vi "Get Package Installed Version.vi"(8 "error in":errorcluster, 11 "package name":string) -> (0 "error out":errorcluster, 1 "installed?":bool, 2 "installed version":string, 3 "package name out":string)   [LabVIEW 2014, in "NIPM_API.lvlib"]
doc: "Returns the version of the package that is currently installed.\n\nINPUT(s)\n<B>Package name</B>: Specifies the package\n\nOUTPUT(s)\n<B>Package name out</B>: Outputs the package name\n\n<B>Installed version</B>: Outputs the currently installed version of the package\n\n<B>Installed?</B>: Outputs whether or not the package is currently installed"
uses:
  NIPM_API.lvlib
panel:
  out "cmd standard output":string
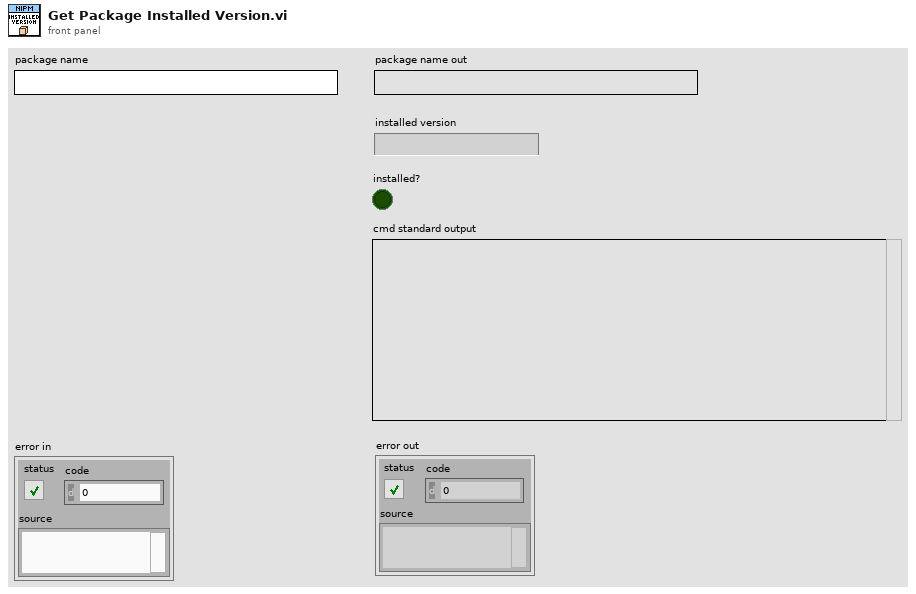
[diagram p1: front panel]
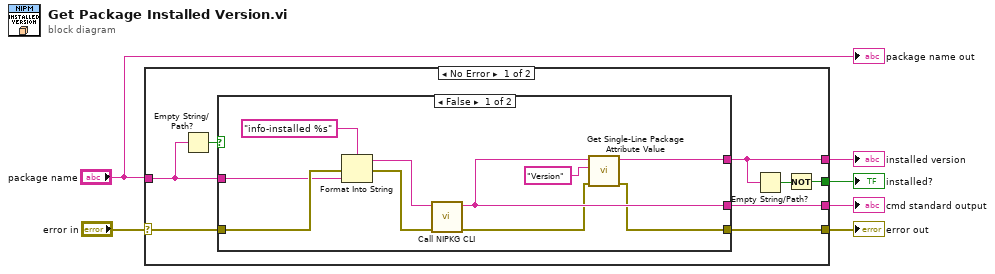
[diagram p0: block diagram]
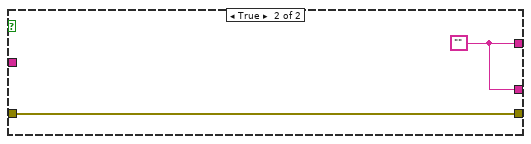
[diagram p2: hidden frame]
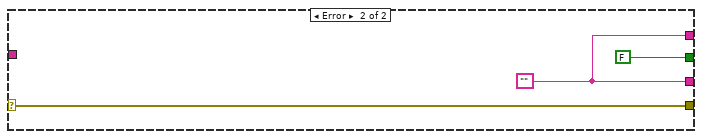
[diagram p3: hidden frame]
diagram:
  n1 = case shown="No Error" "error in" {
    selector: "error in" -> [w14 w29]
    tunnel: [w13 w28] -> w5
    tunnel: [w12 w29] -> w4
    tunnel: "package name" -> [w11 _]
    tunnel: [w9 w28] -> w2
    tunnel: [w7 FALSE] -> w1
    frame No Error {
      n2 = Empty String/Path?(string/path=w11) -> (empty?=w10:bool)
      n3 = case shown="False" w10 {
        tunnel: w14 -> [w23 w26]
        tunnel: [w20 w25] -> w13
        tunnel: [w18 w25] -> w9
        tunnel: [w16 w26] -> w12
        tunnel: w11 -> [w15 _]
        frame False {
          n4 = Format Into String(format string="info-installed %s", error in=w23, w15) -> (resulting string=w22:string, error out=w21:errorcluster)  [unwired: 1 in]
          n5 = call "Call NIPKG CLI.vi"("error in (no error)"=w21, "command"=w22) -> ("error out"=w17:errorcluster, "command line standard output"=w20:string)  [unwired: 8 in]
          n6 = call "Get Single-Line Package Attribute Value.vi"("error in (no error)"=w17, "package attribute name"="Version", "package attributes CLI string"=w20) -> ("error out"=w16:errorcluster, "package attribute value"=w18:string)  [unwired: 6 in, 1 out]
        }
        frame True {
          w25 = ""
        }
      }
      n7 = Empty String/Path?(string/path=w9) -> (empty?=w8:bool)
      n8 = Not(x=w8) -> (.not. x?=w7:bool)
    }
    frame Error {
      w28 = "" ("standard output")
    }
  }
  "error out" <- w4
  "cmd standard output" <- w5
  "installed version" <- w2
  "installed?" <- w1
  "package name out" <- "package name"
